vi "Configure FM Internal [FM].vi"(7 "modulation waveform (Sine)":i32(ring)=1 items=["Sine"=1, "Square"=2, "Triangle"=3, "Ramp Up"=4, "Ramp Down"=5], 8 "error in (no error)":errorcluster, 9 "modulation frequency (1000 Hz)":dbl[unit]=1000.0 format="%^.2e", 10 "peak deviation (100 Hz)":dbl[unit]=100.0 format="%^.2e", 11 "CS++Fgen in":refnum<class "CS++Fgen.lvclass">) -> (0 "error out":errorcluster, 3 "CS++Fgen out":refnum<class "CS++Fgen.lvclass">)   [LabVIEW 2015, in "CS++Fgen.lvlib" / "CS++Fgen.lvclass"]
doc: "This VI configures the properties that control the function generator's internal frequency modulation source. These properties are the peak deviation, waveform, and frequency.\n\nNotes:\n\n(1) This VI is part of the IviFgenModulateFM [FM] extension group."
uses:
  CS++Fgen.lvclass
  CSPP_Core/Classes/CS++ProcessVariables/ProcessVariable/PV.lvclass
  PV-Enum.ctl
  CSPP_Core/Classes/CS++ProcessVariables/ProcessVariable/PV.lvclass/PV.ctl
  CS++Fgen.lvclass/CS++Fgen.ctl
  CSPP_Core/Classes/CS++ProcessVariables/ProcessVariable/Write Data.vi
  CSPP_Core/Classes/CS++ProcessVariables/ProcessVariable/Write Timestamp.vi
  CSPP_Core/Classes/CS++ProcessVariables/ProcessVariable/Write Quality.vi
  CSPP_Core/Classes/CS++ProcessVariables/ProcessVariable/Write status.vi
  CSPP_Core/Classes/CS++ProcessVariables/PVConnection/PVConnection.lvclass
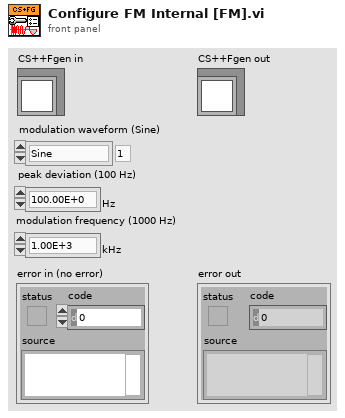
[diagram p1: front panel]
types:
  T1 = typedef "CS++Fgen.lvlib/CS++Fgen.lvclass/PV-Enum.ctl" = enum16{"AM-ModulationDepth", "AM-ModulationFrequency", "FM-ModulationFrequency", "FP-PeakDeviation", "SampleRate", "TriggerRate", "AM-ModulationWaveform", "FM-ModulationWaveform", "OutputMode", "ReferenceClockSource", "SampleClockSource", "SampleClockOutputEnabled"}
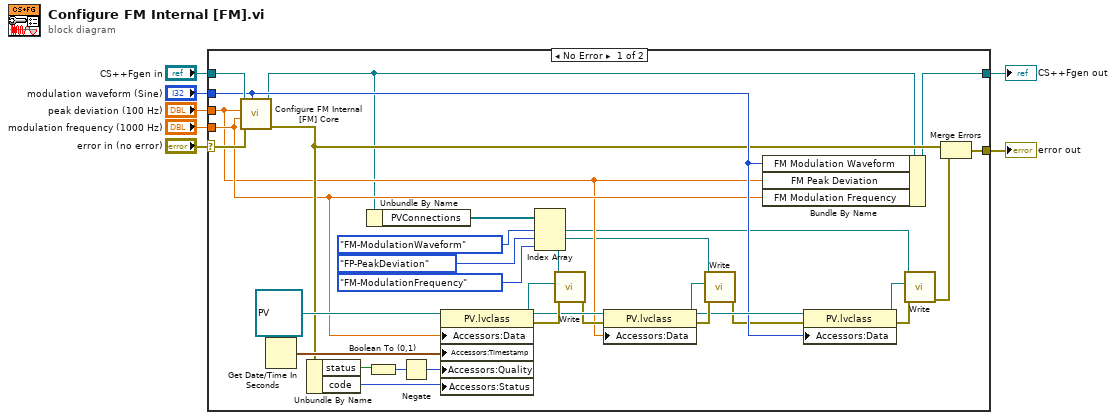
[diagram p0: block diagram]
diagram:
  n1 = case shown="No Error" "error in (no error)" {
    selector: "error in (no error)" -> [w37 w40]
    tunnel: [w22 w40] -> w6
    tunnel: [w16 w39] -> w4
    tunnel: "CS++Fgen in" -> [w38 w39]
    tunnel: "modulation waveform (Sine)" -> [w21 _]
    tunnel: "peak deviation (100 Hz)" -> [w18 _]
    tunnel: "modulation frequency (1000 Hz)" -> [w19 _]
    frame No Error {
      n2 = call-dynamic "Configure FM Internal [FM] Core.vi"("modulation waveform (Sine)"=w21, "error in (no error)"=w37, "modulation frequency (1000 Hz)"=w19, "peak deviation (100 Hz)"=w18, "CS++Fgen in"=w38) -> ("error out"=w20:errorcluster, "CS++Fgen out"=w17:refnum<class "CS++Fgen.lvclass">)  [unwired: 5 in]
      n3 = Get Date/Time In Seconds() -> (seconds since 1Jan1904=w36:timestamp)
      n4 = Unbundle By Name(w20) -> ("status"=w33:bool, "code"=w31:i32)
      n5 = Unbundle By Name(w17) -> ("PVConnections"=w14:refnum<class "PVConnection.lvclass">[])
      n6 = Boolean To (0,1)(Boolean=w33) -> (0, 1=w32:i16)
      n7 = Negate(x=w32) -> (-x=w30:i16)
      n8 = property class="PV.lvclass"(reference=refnum<class "PV.lvclass"> refnum ("PV"), "Accessors:Data"=w19, "Accessors:Timestamp"=w36, "Accessors:Quality"=w30, "Accessors:Status"=w31) -> (reference out=w28:refnum<class "PV.lvclass">, error out=w34:errorcluster)  [unwired: 1 in]
      n9 = Index Array(array=w14, index #1=PV-Enum."FM-ModulationWaveform" ("PV-Enum"), index #2=PV-Enum."FP-PeakDeviation" ("PV-Enum"), index #3=PV-Enum."FM-ModulationFrequency" ("PV-Enum")) -> (element #1=w13:refnum<class "PVConnection.lvclass">, element #2=w11:refnum<class "PVConnection.lvclass">, element #3=w12:refnum<class "PVConnection.lvclass">)
      n10 = call "Write.vi"("error in (no error)"=w34, "PV"=w28, "PVConnection in"=w12) -> ("error out"=w27:errorcluster)  [unwired: 7 in, 1 out]
      n11 = property class="PV.lvclass"(reference=w28, error in=w27, "Accessors:Data"=w18) -> (reference out=w24:refnum<class "PV.lvclass">, error out=w29:errorcluster)
      n12 = call "Write.vi"("error in (no error)"=w29, "PV"=w24, "PVConnection in"=w11) -> ("error out"=w15:errorcluster)  [unwired: 7 in, 1 out]
      n13 = Bundle By Name(cluster=w17, "FM Modulation Waveform"=w21, "FM Peak Deviation"=w18, "FM Modulation Frequency"=w19) -> (w16:refnum<class "CS++Fgen.lvclass">)
      n14 = property class="PV.lvclass"(reference=w24, error in=w15, "Accessors:Data"=w21) -> (reference out=w25:refnum<class "PV.lvclass">, error out=w26:errorcluster)
      n15 = call "Write.vi"("error in (no error)"=w26, "PV"=w25, "PVConnection in"=w13) -> ("error out"=w23:errorcluster)  [unwired: 7 in, 1 out]
      n16 = Merge Errors(w20, w23) -> (w22:errorcluster)
    }
    frame Error {
    }
  }
  "error out" <- w6
  "CS++Fgen out" <- w4
